vi "TMP36.vi"(7 "Analog Ref Override":dbl, 8 "Error In":errorcluster, 10 "Analog Channel":u8, 11 "LINX Resource":T1) -> (0 "Error Out":errorcluster, 2 "Temp C":dbl, 3 "LINX Resource":T1)   [LabVIEW 2013, in "LVH-LINX.lvlib" / "TMP3x.lvlib"]
doc: "Read temperature from TMP36"
uses:
  <vilib>/LabVIEW Hacker/LINX/Public/Sensors/Temperature/TMP3x/TMP3x.lvlib
  <vilib>/LabVIEW Hacker/LINX/Private/Type Defs/LINX Ref.ctl
  <vilib>/LabVIEW Hacker/LINX/Private/Type Defs/Platform.ctl
  <vilib>/LabVIEW Hacker/LINX/Private/Type Defs/Interface.ctl
  <vilib>/LabVIEW Hacker/LINX/Private/Device/Type Defs/LINX Device Config.ctl
  <vilib>/LabVIEW Hacker/LINX/Private/Device/Type Defs/TCP Config.ctl
  <vilib>/LabVIEW Hacker/LINX/Private/Type Defs/Device Family.ctl
  <vilib>/LabVIEW Hacker/LINX/Public/Peripherals/Analog/Analog Read 1 Chan.vi
  <vilib>/LabVIEW Hacker/LINX/LVH-LINX.lvlib
  <vilib>/LabVIEW Hacker/LINX/Private/Device/Device.lvlib
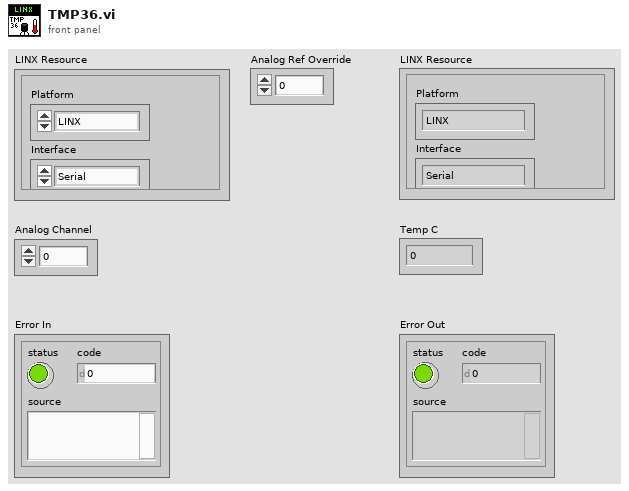
[diagram p1: front panel]
types:
  T1 = typedef "LVH-LINX.lvlib/LINX Ref.ctl" = cluster{"Platform":T2, "Interface":T3, "LINX Device Config":T4}
  T2 = typedef "LVH-LINX.lvlib/Platform.ctl" = enum16{"LINX", "myRIO"}
  T3 = typedef "LVH-LINX.lvlib/Interface.ctl" = enum16{"Serial", "TCP"}
  T4 = typedef "LVH-LINX.lvlib/Device.lvlib/LINX Device Config.ctl" = cluster{"Interface":T3, "COM Port":refnum<visa-resource-name>, "TCP Configuration":T5, "Device Family":T6, "Device ID":u8, "Device Name":string, "TCP Ref":refnum<k5>}
  T5 = typedef "LVH-LINX.lvlib/Device.lvlib/TCP Config.ctl" = cluster{"IP Address":string, "Port":u16}
  T6 = typedef "LVH-LINX.lvlib/Device Family.ctl" = enum8{"National Instruments", "Digilent", "Arduino"}
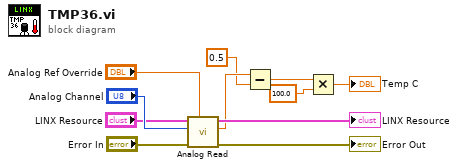
[diagram p0: block diagram]
diagram:
  n1 = call-poly <vilib>:"Analog Read.vi"("Analog Ref Override"="Analog Ref Override", "Error In"="Error In", "Analog Channel"="Analog Channel", "LINX Resource"="LINX Resource") -> ("Error Out"=→"Error Out":errorcluster, "AI Value"=w2:dbl, "LINX Resource"=→"LINX Resource":T1)  [unwired: 4 in, 1 out]
  n2 = Subtract(x=w2, y=0.5) -> (x-y=w3:dbl)
  n3 = Multiply(x=w3, y=100.0) -> (x*y=→"Temp C":dbl)
